vi "Sensorarray_aufloesen.vi"(2 "Array":dbl[](array[numeric])) -> (11 "hinten links":dbl, 13 "hinten rechts":dbl, 14 "vorne rechts":dbl, 15 "vorne links":dbl, 16 "schräg rechts":dbl, 17 "schräg links":dbl, 18 "gerade rechts":dbl, 19 "gerade links":dbl)   [LabVIEW 2016]
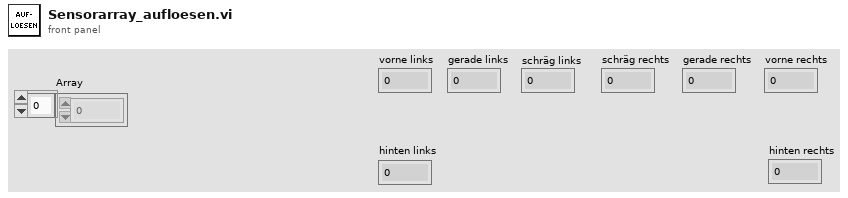
[diagram p1: front panel]
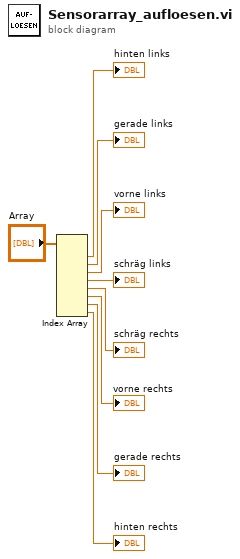
[diagram p0: block diagram]
diagram:
  n1 = Index Array(array="Array") -> (element #1=→"hinten links":dbl, element #2=→"gerade links":dbl, element #3=→"vorne links":dbl, element #4=→"schräg links":dbl, element #5=→"schräg rechts":dbl, element #6=→"vorne rechts":dbl, element #7=→"gerade rechts":dbl, element #8=→"hinten rechts":dbl)  [unwired: 8 in]
